vi "VD-unsetUSBMode.vi"(8 "error in (no error)":errorcluster, 11 "VD-LV-LiteVNA in":refnum<class "VD-LV-LiteVNA.lvclass">) -> (0 "error out":errorcluster, 3 "VD-LV-LiteVNA out":refnum<class "VD-LV-LiteVNA.lvclass">)   [LabVIEW 2020, in "VD-LV-LiteVNA.lvclass"]
uses:
  VD-LV-LiteVNA.lvclass
  VD-action.ctl
  VD-LV-LiteVNA.lvclass/VD-LV-LiteVNA.ctl
  hardware-protocol/serial/HP-S-Serial.lvclass
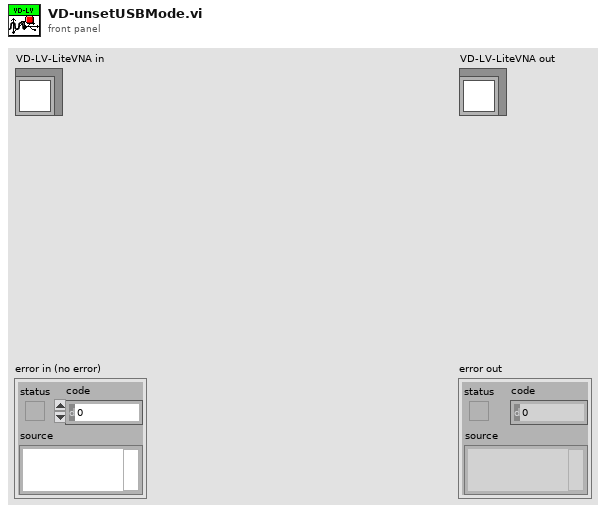
[diagram p1: front panel]
types:
  T1 = typedef "VD-LV-LiteVNA.lvclass/VD-action.ctl" = enum16{"checkCom", "SweepStartHz", "SweepStopHz", "SweepPoints", "valuesPerFrequency", "RawSamplesMode", "ValuesFIFO", "deviceVariant", "protocolVersion", "hardwareRevision", "firmwareMajor", "firmwareMinor"}
  T2 = typedef "HP-S-Serial.lvclass/HP-S-data.ctl" = u8[]
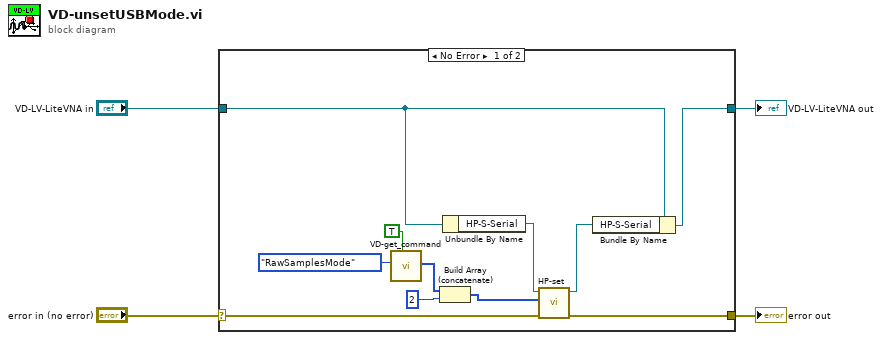
[diagram p0: block diagram]
diagram:
  n1 = case shown="No Error" "error in (no error)" {
    selector: "error in (no error)" -> [w6 w17]
    tunnel: [w5 w17] -> w3
    tunnel: [w9 w16] -> w1
    tunnel: "VD-LV-LiteVNA in" -> [w8 w16]
    frame No Error {
      n2 = call "VD-get_command.vi"("Write?"=TRUE, "action"=VD-action."RawSamplesMode") -> ("Command"=w13:T2)  [unwired: 9 in]
      n3 = Build Array (concatenate)(w13, u8 2 ("8bit")) -> (w10:T2)
      n4 = Unbundle By Name(w8) -> ("HP-S-Serial"=w15:refnum<class "HP-S-Serial.lvclass">)
      n5 = call-dynamic "HP-set.vi"("error in (no error)"=w6, "write buffer"=w10, "HP-S-Serial in"=w15) -> ("error out"=w5:errorcluster, "HP-S-Serial out"=w14:refnum<class "HP-S-Serial.lvclass">)  [unwired: 7 in]
      n6 = Bundle By Name(cluster=w8, "HP-S-Serial"=w14) -> (w9:refnum<class "VD-LV-LiteVNA.lvclass">)
    }
    frame Error {
    }
  }
  "error out" <- w3
  "VD-LV-LiteVNA out" <- w1
